vi "Analogs.vi"() -> ()   [LabVIEW 2016]
uses:
  controls/EnumFGVHDT.ctl
  controls/Enum.ctl
  Course Project/support/Message Queue/Message Cluster.ctl
  <vilib>/rvi/errors/niLvFpgaAdjustHostInterfaceError.vi
  controls/FPGAVIreferenceTypeDef.ctl
  <vilib>/rvi/interface/nirviReadWriteControl/nirviReadWriteControl.xnode
  FPGA Bitfiles/lbniAFMControlle_flexRio_controllerFPGA.lvbitx
  <vilib>/regexp/Match Regular Expression.xnode
  NiFpgaLv.dll
  Course Project/support/Message Queue/Message Queue.lvlib
panel:
  in  "Analog Inputs":T1
  in  "Analog Outputs":T2
  # "Inverted"
  # "Non Inverted"
  # "Inverted"
  # "Non inverted"
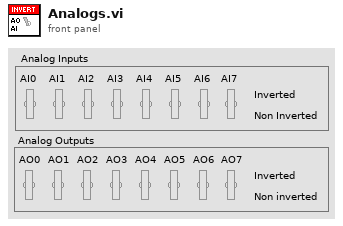
[diagram p1: front panel]
types:
  T1 = cluster{"AI0":bool, "AI1":bool, "AI2":bool, "AI3":bool, "AI4":bool, "AI5":bool, "AI6":bool, "AI7":bool}
  T2 = cluster{"AO0":bool, "AO1":bool, "AO2":bool, "AO3":bool, "AO4":bool, "AO5":bool, "AO6":bool, "AO7":bool}
  T3 = typedef "EnumFGVHDT.ctl" = enum16{"Init", "Read", "Write", "Push", "Pop"}
  T4 = typedef "Message Queue.lvlib/All Message Queues.ctl" = cluster{"IU":refnum<queue>}
  T5 = typedef "Message Queue.lvlib/Message Cluster.ctl" = cluster{"Message":string, "Données de message":variant}
  T6 = typedef "Enum.ctl" = enum16{"Init", "Read", "Write"}
  T7 = typedef "FPGAVIreferenceTypeDef.ctl" = refnum<k20>
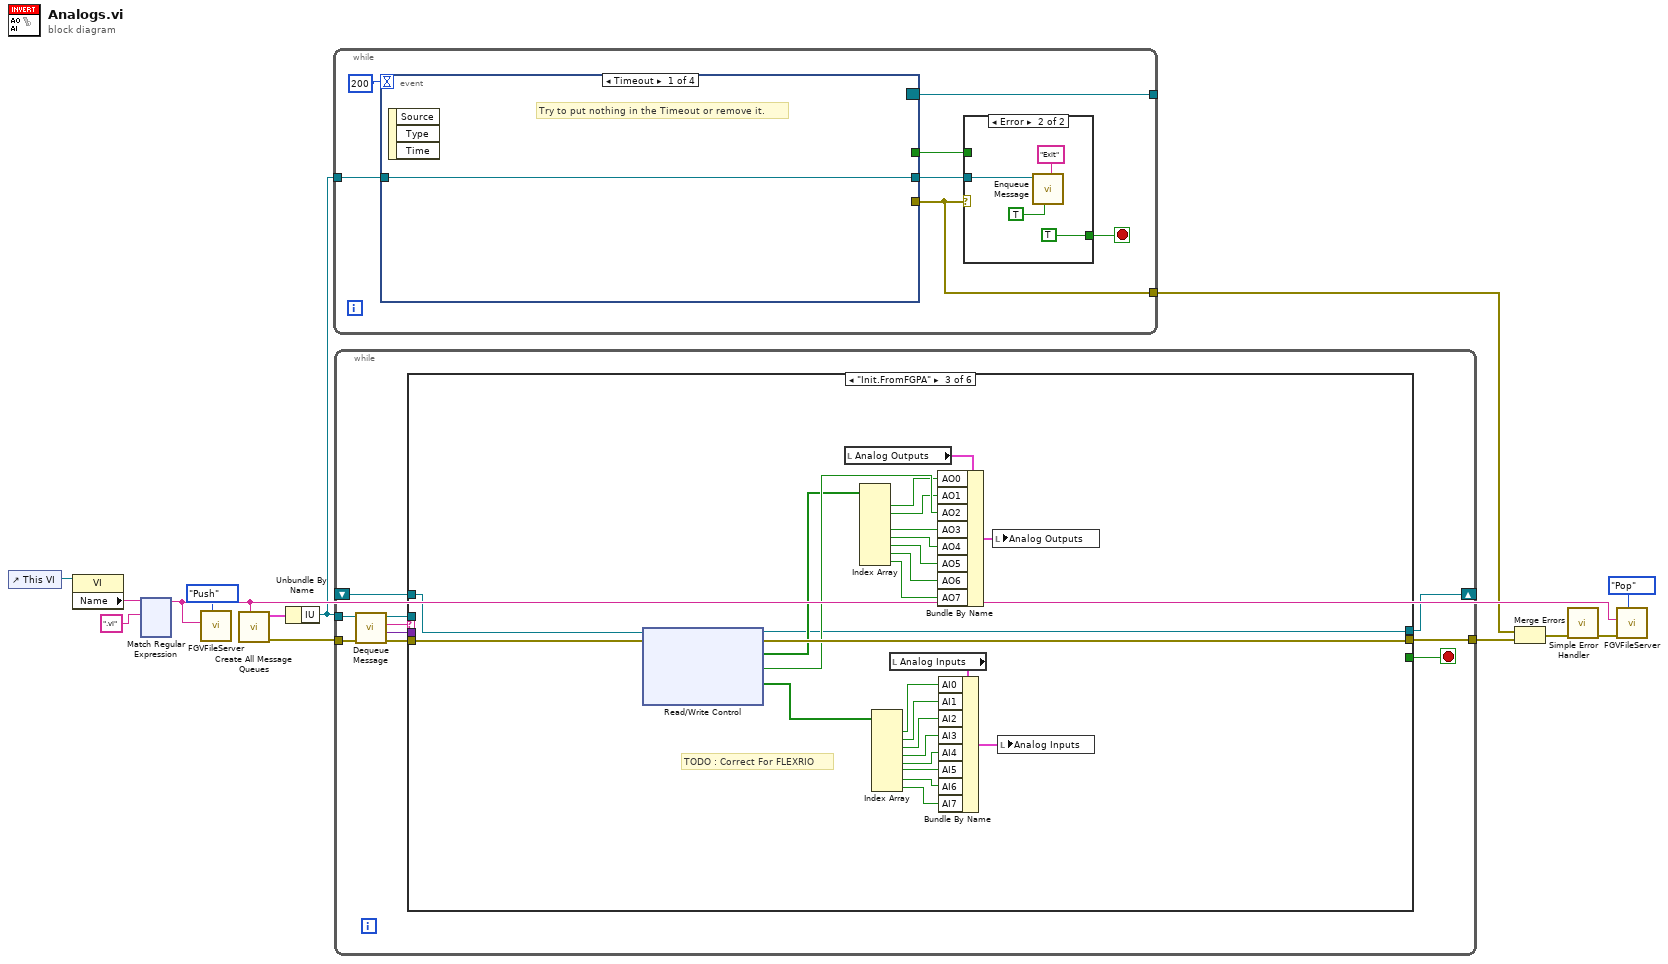
[diagram p0: block diagram]
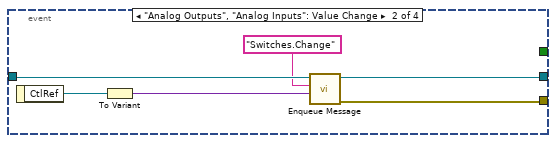
[diagram p3: hidden frame]
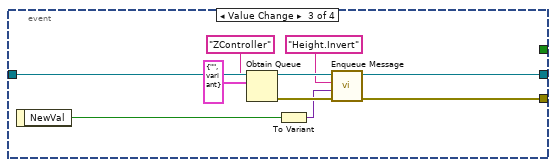
[diagram p4: hidden frame]
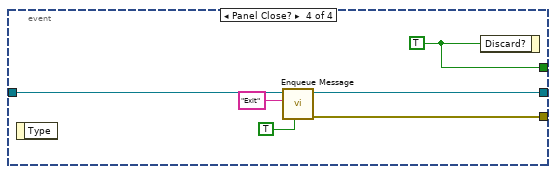
[diagram p5: hidden frame]
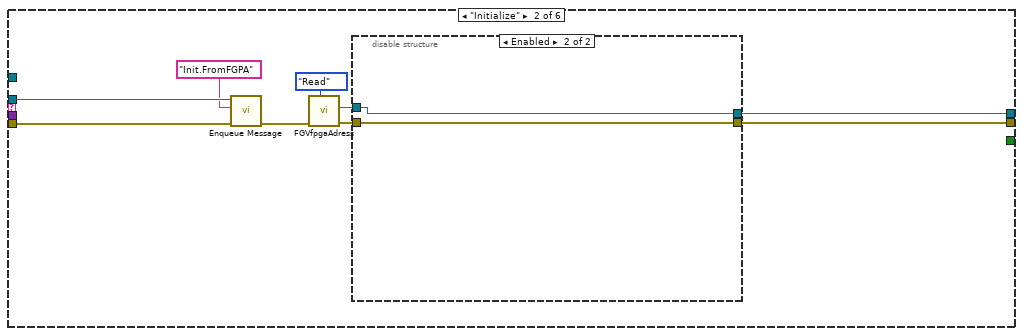
[diagram p7: hidden frame]
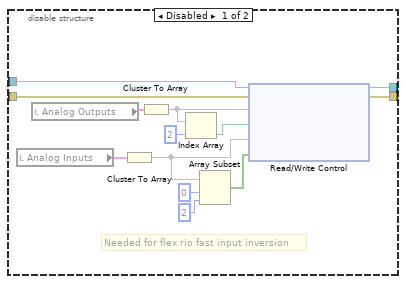
[diagram p8: hidden frame]
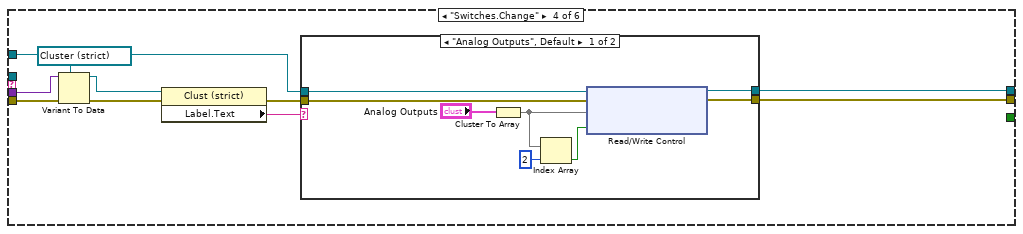
[diagram p9: hidden frame]
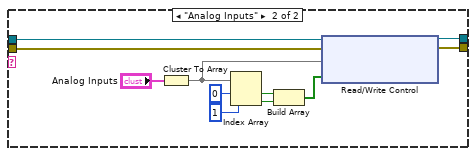
[diagram p10: hidden frame]
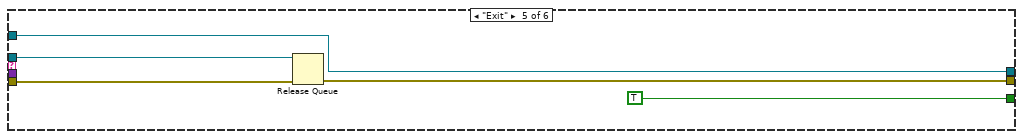
[diagram p11: hidden frame]
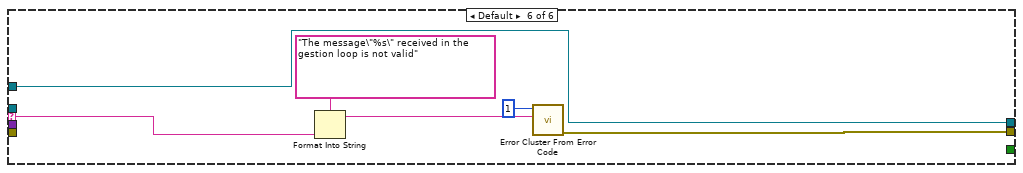
[diagram p12: hidden frame]
diagram:
  n1 = control-ref of="This VI"() -> (w12:refnum<vi>)
  n2 = property class="VI"(reference=w12) -> ("Name"=w11:string)  [unwired: 1 in, 2 out]
  n3 = xnode "Match Regular Expression"("input string"=w11, "regular expression"=".vi") -> ("before match"=w13:string)  [unwired: 4 in, 4 out]
  n4 = call "FGVFileServer.vi"("Enum"=EnumFGVHDT."Push", "New VI"=w13) -> ()  [unwired: 8 in, 2 out]
  n5 = call "Create All Message Queues.vi"("QueueName"=w13) -> ("ErrorOut"=w7:errorcluster, "MessageQueueOut"=w9:T4)  [unwired: 9 in]
  n6 = Unbundle By Name(w9) -> ("IU"=w8:refnum<queue>)
  n7 = while {
    tunnel: w8 -> [w20]
    tunnel: [w16] -> w4
    tunnel: [w15] -> _
    stop <- w18 stop-if-true
    n8 = event shown="[0] Timeout" {
      selector: _ -> [_ _ _ _]
      dyn-events: [_ _ _ _] -> w15
      timeout: 200 -> [_ _ _ _]
      tunnel: [_ _ _ w47] -> w19
      tunnel: w20 -> [w26 w32 w40 w46]
      tunnel: [_ w30 w34 w45] -> w16
      tunnel: [w26 w31 w40 w44] -> w17
      event Timeout {
        # "Try to put nothing in the Timeout or remove it."
        n9 = event-data() -> ()  [unwired: 1 in, 3 out]
      }
      event "Analog Outputs", "Analog Inputs": Value Change {
        n10 = event-data() -> ("CtlRef"=w29:refnum<vi>)  [unwired: 1 in]
        n11 = To Variant(anything=w29) -> (Variant=w28:variant)
        n12 = call "Enqueue Message.vi"("Data"=w28, "Message"="Switches.Change", "Queue"=w32) -> ("error out"=w30:errorcluster, "Queue dup."=w31:refnum<queue>)  [unwired: 7 in]
      }
      event "Analog Outputs.AO2": Value Change {
        n13 = event-data() -> ("NewVal"=w33:bool)  [unwired: 1 in]
        n14 = Obtain Queue(name (unnamed)="ZController" ("QueueName"), element data type=T5 {"Message"="", "Données de message"=variant} ("Cluster Message")) -> (queue out=w39:refnum<queue>, error out=w41:errorcluster)  [unwired: 3 in, 1 out]
        n15 = To Variant(anything=w33) -> (Variant=w38:variant)
        n16 = call "Enqueue Message.vi"("error in"=w41, "Data"=w38, "Message"="Height.Invert", "Queue"=w39) -> ("error out"=w34:errorcluster)  [unwired: 6 in, 1 out]
      }
      event Panel Close? {
        w47 = TRUE ("Rejeter ?")
        n17 = event-data() -> ()  [unwired: 1 in, 1 out]
        n18 = call "Enqueue Message.vi"("Prioritary message"=TRUE ("Message prioritaire ? (F)"), "Message"="Exit", "Queue"=w46) -> ("error out"=w45:errorcluster, "Queue dup."=w44:refnum<queue>)  [unwired: 7 in]
        n19 = event-data ("Event Filter Node")("Discard?"=w47) -> ()  [unwired: 1 in, 1 out]
      }
    }
    n20 = case shown="Error" w16 {
      tunnel: [w21 TRUE ("Rejeter ?")] -> w18
      tunnel: w19 -> [w21 _]
      tunnel: w17 -> [_ w24]
      frame No Error {
      }
      frame Error {
        n21 = call "Enqueue Message.vi"("Prioritary message"=TRUE ("Message prioritaire ? (F)"), "Message"="Exit", "Queue"=w24) -> ()  [unwired: 7 in, 2 out]
      }
    }
  }
  n22 = while {
    tunnel: w8 -> [w51]
    tunnel: w7 -> [w55]
    tunnel: [w56] -> w5
    shift-right: [w49] -> _
    shift-left: _ -> [w48]
    stop <- w57 stop-if-true
    n23 = call "Dequeue Message.vi"("entrée d'erreur (pas d'erreur)"=w55, "File d'attente de messages"=w51) -> ("sortie d'erreur"=w54:errorcluster, "Données de message"=w53:variant, "Message"=w50:string, "File d'attente de message dup."=w52:refnum<queue>)  [unwired: 6 in]
    n24 = case "Conditions des messages" shown="\"Init.FromFGPA\"" w50 {
      selector: w50 -> [_ _ _ _ _ w148]
      tunnel: w52 -> [_ w68 _ _ w143 _]
      tunnel: w54 -> [w59 w61 w85 w116 w141 _]
      tunnel: [w59 w62 w109 w117 w140 w146] -> w56
      tunnel: [_ _ _ _ TRUE _] -> w57
      tunnel: w53 -> [_ _ _ w113 _ _]
      tunnel: [w58 w66 w86 w118 w139 w144] -> w49
      tunnel: w48 -> [w58 _ w84 w111 w139 w144]
      frame "--------- Initialization ---------" {
      }
      frame "Initialize" {
        n25 = call "Enqueue Message.vi"("error in"=w61, "Message"="Init.FromFGPA", "Queue"=w68) -> ("error out"=w60:errorcluster)  [unwired: 7 in, 1 out]
        n26 = call "FGVfpgaAdress.vi"("Enum"=Enum."Read", "error in"=w60) -> ("error out"=w65:errorcluster, "FPGA VI Reference Out"=w64:T7)  [unwired: 4 in, 4 out]
        n27 = disable-structure shown="Enabled" {
          disable-tunnel: [w72 w83] -> w66
          disable-tunnel: w65 -> [w71 w82]
          disable-tunnel: w64 -> [w70 w83]
          disable-tunnel: [w69 w82] -> w62
          frame Disabled {
            # "Needed for flex rio fast input inversion"
            n28 = local read "Analog Inputs"() -> (w73:T1)
            n29 = local read "Analog Outputs"() -> (w74:T2)
            n30 = Cluster To Array(cluster=w73) -> (array=w78:bool[])
            n31 = Cluster To Array(cluster=w74) -> (array=w75:bool[])
            n32 = Index Array(array=w75, index=2) -> (element=w76:bool)
            n33 = Array Subset(array=w78, index=0, length=2) -> (w79:bool[])
            n34 = xnode "Read/Write Control"("FPGA VI Reference In"=w70, "error in"=w71, "aio.o.invertOutputs"=w75, "aio.o.invertHeight"=w76, "aio.o.invertInputs"=w78, "aio.o.invert2Inputs"=w79) -> ("FPGA VI Reference Out"=w72:T7, "error out"=w69:errorcluster)
          }
          frame Enabled {
          }
        }
      }
      frame "Init.FromFGPA" {
        # "TODO : Correct For FLEXRIO"
        n35 = xnode "Read/Write Control"("FPGA VI Reference In"=w84, "error in"=w85) -> ("FPGA VI Reference Out"=w86:T7, "error out"=w109:errorcluster, "aio.o.invertOutputs"=w88:bool[], "aio.o.invertHeight"=w108:bool, "aio.o.invertInputs"=w97:bool[])  [unwired: 1 out]
        n36 = local read "Analog Outputs"() -> (w87:T2)
        n37 = Index Array(array=w88) -> (element #1=w89:bool, element #2=w90:bool, element #4=w91:bool, element #5=w92:bool, element #6=w93:bool, element #7=w94:bool, element #8=w95:bool)  [unwired: 8 in, 1 out]
        n38 = Index Array(array=w97) -> (element #1=w100:bool, element #2=w101:bool, element #3=w102:bool, element #4=w103:bool, element #5=w104:bool, element #6=w105:bool, element #7=w106:bool, element #8=w107:bool)  [unwired: 8 in]
        n39 = local read "Analog Inputs"() -> (w98:T1)
        n40 = Bundle By Name(cluster=w87, "AO0"=w89, "AO1"=w90, "AO2"=w108, "AO3"=w91, "AO4"=w92, "AO5"=w93, "AO6"=w94, "AO7"=w95) -> (w96:T2)
        n41 = Bundle By Name(cluster=w98, "AI0"=w100, "AI1"=w101, "AI2"=w102, "AI3"=w103, "AI4"=w104, "AI5"=w105, "AI6"=w106, "AI7"=w107) -> (w99:T1)
        n42 = local write "Analog Outputs"(w96) -> ()
        n43 = local write "Analog Inputs"(w99) -> ()
      }
      frame "Switches.Change" {
        n44 = Variant To Data(error in=w116, type=refnum<vi> refnum ("CtlRef"), Variant=w113) -> (data=w110:refnum<vi>, error out=w114:errorcluster)
        n45 = property class="Clust (strict)"(reference=w110, error in=w114) -> (error out=w115:errorcluster, "Label.Text"=w119:string)  [unwired: 1 out]
        n46 = case shown="\"Analog Outputs\", Default" w119 {
          tunnel: w111 -> [w127 w138]
          tunnel: [w126 w137] -> w118
          tunnel: w115 -> [w124 w135]
          tunnel: [w120 w128] -> w117
          frame "Analog Outputs", Default {
            n47 = Cluster To Array(cluster="Analog Outputs") -> (array=w123:bool[])
            n48 = Index Array(array=w123, index=2) -> (element=w122:bool)
            n49 = xnode "Read/Write Control"("FPGA VI Reference In"=w127, "error in"=w124, "aio.o.invertOutputs"=w123, "aio.o.invertHeight"=w122) -> ("FPGA VI Reference Out"=w126:T7, "error out"=w120:errorcluster)
          }
          frame "Analog Inputs" {
            n50 = Cluster To Array(cluster="Analog Inputs") -> (array=w134:bool[])
            n51 = Index Array(array=w134, index #1=0 ("index"), index #2=1 ("index")) -> (element #1=w131:bool, element #2=w130:bool)
            n52 = Build Array(w131, w130) -> (w129:bool[])
            n53 = xnode "Read/Write Control"("FPGA VI Reference In"=w138, "error in"=w135, "aio.o.invertInputs"=w134, "aio.o.invert2Inputs"=w129) -> ("FPGA VI Reference Out"=w137:T7, "error out"=w128:errorcluster)
          }
        }
      }
      frame "Exit" {
        n54 = Release Queue(queue=w143, error in (no error)=w141) -> (error out=w140:errorcluster)  [unwired: 1 in, 2 out]
      }
      frame Default {
        n55 = Format Into String(format string="The message\"%s\" received in the gestion loop is not valid" ("Texte de message d'erreur inconnu"), w148) -> (resulting string=w145:string)  [unwired: 2 in, 1 out]
        n56 = call <vilib>:"Error Cluster From Error Code.vi"("error message (\"\")"=w145, "error code (0)"=1 ("code d'erreur (0)")) -> ("error out"=w146:errorcluster)  [unwired: 7 in]
      }
    }
  }
  n57 = Merge Errors(w4, w5) -> (w6:errorcluster)
  n58 = call <vilib>:"Simple Error Handler.vi"("error in (no error)"=w6) -> ("error out"=w2:errorcluster)  [unwired: 4 in, 4 out]
  n59 = call "FGVFileServer.vi"("Enum"=EnumFGVHDT."Pop", "error in"=w2, "New VI"=w13) -> ()  [unwired: 7 in, 2 out]
